vi "VI Tree.vi"   [LabVIEW 2015, in "IT6000C.lvlib"]
doc: "This is the instrument driver for the <INSTRUMENT NAME>. The VI Tree displays all the user-callable VIs of the instrument driver in an organized table."
uses:
  <instrlib>/IT6000C/IT6000C.lvlib
panel:
  # "(c) 2014 <Enter Company Name Here>.  ALL RIGHTS RESERVED."
  # "SEE DIAGRAM\nFOR VI TREE."
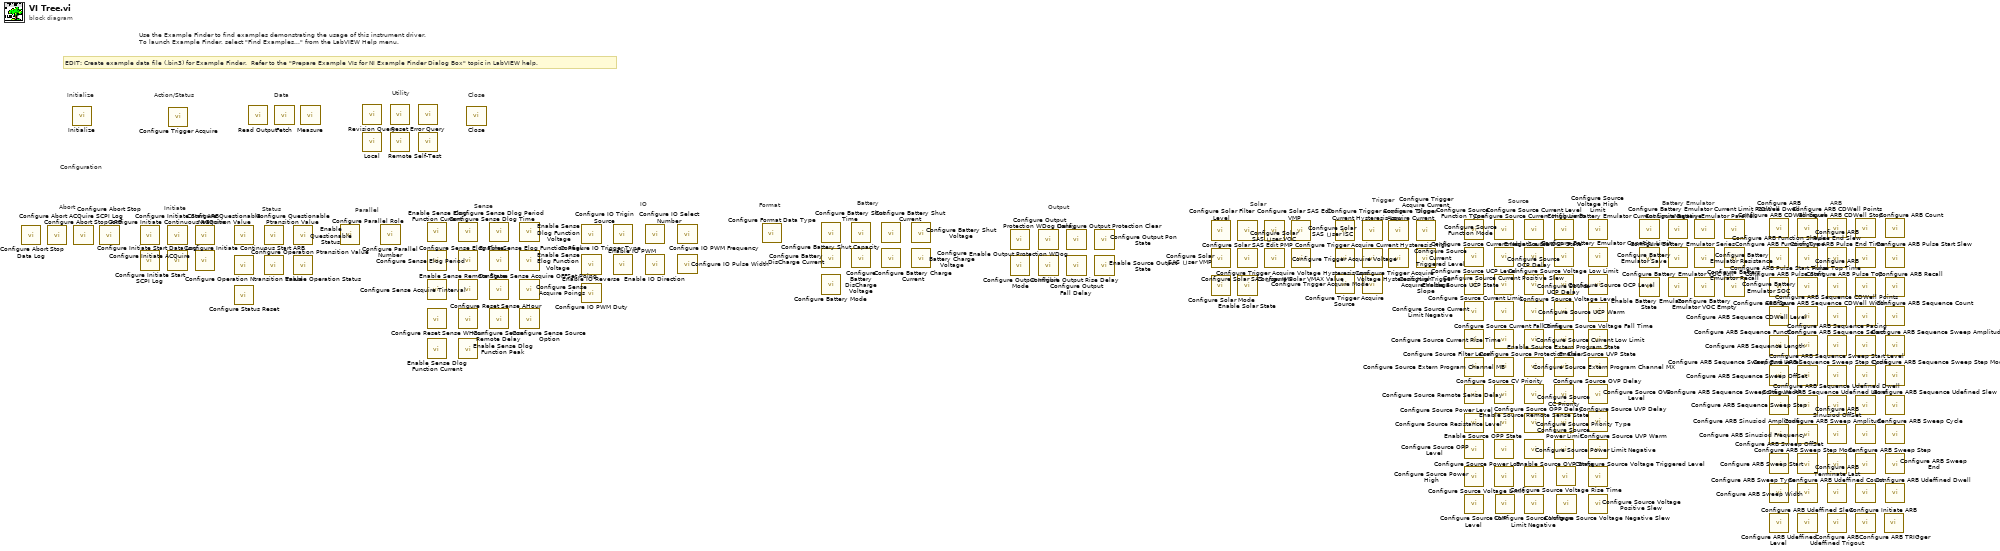
[diagram p0: block diagram]
diagram:
  # "Output"
  # "ARB"
  # "Battery Emulator"
  # "Source"
  # "Trigger"
  # "Solar"
  # "Battery"
  # "Format"
  # "IO"
  # "Sense"
  # "Parallel"
  # "Status"
  # "Initiate"
  # "Abort"
  # "EDIT: Create example data file (.bin3) for Example Finder.  Refer to the \"Prepare Example VIs for NI Example Finder Dialog Box\" topic in LabVIEW help."
  # "Use the Example Finder to find examples demonstrating the usage of this instrument driver.\nTo launch Example Finder, select \"Find Examples...\" from the LabVIEW Help menu."
  # "Configuration"
  # "Utility"
  # "Data"
  # "Action/Status"
  # "Close"
  # "Initialize"
  n1 = call <instrlib>:"Configure Abort Stop Data Log.vi"() -> ()  [unwired: 10 in, 2 out]
  n2 = call <instrlib>:"Configure Abort ACQuire.vi"() -> ()  [unwired: 10 in, 2 out]
  n3 = call <instrlib>:"Initialize.vi"() -> ()  [unwired: 10 in, 2 out]
  n4 = call <instrlib>:"Configure Abort Stop ARB.vi"() -> ()  [unwired: 10 in, 2 out]
  n5 = call <instrlib>:"Configure Abort Stop SCPI Log.vi"() -> ()  [unwired: 10 in, 2 out]
  n6 = call <instrlib>:"Configure Initiate ACQuire.vi"() -> ()  [unwired: 10 in, 2 out]
  n7 = call <instrlib>:"Configure Initiate Start SCPI Log.vi"() -> ()  [unwired: 10 in, 2 out]
  n8 = call <instrlib>:"Configure Initiate Start ARB.vi"() -> ()  [unwired: 10 in, 2 out]
  n9 = call <instrlib>:"Configure Initiate Start Data Log.vi"() -> ()  [unwired: 10 in, 2 out]
  n10 = call <instrlib>:"Configure Trigger Acquire.vi"() -> ()  [unwired: 10 in, 2 out]
  n11 = call <instrlib>:"Configure Initiate Continuous ACQuire.vi"() -> ()  [unwired: 10 in, 2 out]
  n12 = call <instrlib>:"Configure Initiate Continuous Start ARB.vi"() -> ()  [unwired: 10 in, 2 out]
  n13 = call <instrlib>:"Configure Questionable Ntransition Value.vi"() -> ()  [unwired: 10 in, 2 out]
  n14 = call <instrlib>:"Configure Operation Ntransition Value.vi"() -> ()  [unwired: 10 in, 2 out]
  n15 = call <instrlib>:"Configure Status Reset.vi"() -> ()  [unwired: 10 in, 2 out]
  n16 = call <instrlib>:"Read Output.vi"() -> ()  [unwired: 8 in, 4 out]
  n17 = call <instrlib>:"Configure Questionable Ptransition Value.vi"() -> ()  [unwired: 10 in, 2 out]
  n18 = call <instrlib>:"Configure Operation Ptransition Value.vi"() -> ()  [unwired: 10 in, 2 out]
  n19 = call <instrlib>:"Fetch.vi"() -> ()  [unwired: 9 in, 3 out]
  n20 = call <instrlib>:"Enable Questionable Status.vi"() -> ()  [unwired: 10 in, 2 out]
  n21 = call <instrlib>:"Enable Operation Status.vi"() -> ()  [unwired: 10 in, 2 out]
  n22 = call <instrlib>:"Measure.vi"() -> ()  [unwired: 9 in, 3 out]
  n23 = call <instrlib>:"Configure Parallel Role.vi"() -> ()  [unwired: 10 in, 2 out]
  n24 = call <instrlib>:"Revision Query.vi"() -> ()  [unwired: 8 in, 4 out]
  n25 = call <instrlib>:"Local.vi"() -> ()  [unwired: 10 in, 2 out]
  n26 = call <instrlib>:"Configure Parallel Number.vi"() -> ()  [unwired: 10 in, 2 out]
  n27 = call <instrlib>:"Reset.vi"() -> ()  [unwired: 10 in, 2 out]
  n28 = call <instrlib>:"Remote.vi"() -> ()  [unwired: 10 in, 2 out]
  n29 = call <instrlib>:"Error Query.vi"() -> ()  [unwired: 8 in, 4 out]
  n30 = call <instrlib>:"Self-Test.vi"() -> ()  [unwired: 8 in, 4 out]
  n31 = call <instrlib>:"Enable Sense Elog Function Current.vi"() -> ()  [unwired: 10 in, 2 out]
  n32 = call <instrlib>:"Configure Sense Elog Time.vi"() -> ()  [unwired: 10 in, 2 out]
  n33 = call <instrlib>:"Enable Sense Remote State.vi"() -> ()  [unwired: 10 in, 2 out]
  n34 = call <instrlib>:"Configure Reset Sense WHour.vi"() -> ()  [unwired: 10 in, 2 out]
  n35 = call <instrlib>:"Enable Sense Dlog Function Current.vi"() -> ()  [unwired: 10 in, 2 out]
  n36 = call <instrlib>:"Configure Sense Dlog Time.vi"() -> ()  [unwired: 10 in, 2 out]
  n37 = call <instrlib>:"Configure Sense Elog Period.vi"() -> ()  [unwired: 10 in, 2 out]
  n38 = call <instrlib>:"Configure Sense Acquire Tinterval.vi"() -> ()  [unwired: 10 in, 2 out]
  n39 = call <instrlib>:"Configure Reset Sense AHour.vi"() -> ()  [unwired: 10 in, 2 out]
  n40 = call <instrlib>:"Enable Sense Dlog Function Peak.vi"() -> ()  [unwired: 10 in, 2 out]
  n41 = call <instrlib>:"Close.vi"() -> ()  [unwired: 11 in, 1 out]
  n42 = call <instrlib>:"Configure Sense Dlog Period.vi"() -> ()  [unwired: 10 in, 2 out]
  n43 = call <instrlib>:"Enable Sense Elog Function Peak.vi"() -> ()  [unwired: 10 in, 2 out]
  n44 = call <instrlib>:"Configure Sense Acquire OFFSet Poing.vi"() -> ()  [unwired: 10 in, 2 out]
  n45 = call <instrlib>:"Configure Sense Remote Delay.vi"() -> ()  [unwired: 10 in, 2 out]
  n46 = call <instrlib>:"Enable Sense Dlog Function Voltage.vi"() -> ()  [unwired: 10 in, 2 out]
  n47 = call <instrlib>:"Enable Sense Elog Function Voltage.vi"() -> ()  [unwired: 10 in, 2 out]
  n48 = call <instrlib>:"Configure Sense Acquire Poings.vi"() -> ()  [unwired: 10 in, 2 out]
  n49 = call <instrlib>:"Configure Sense Source Option.vi"() -> ()  [unwired: 10 in, 2 out]
  n50 = call <instrlib>:"Configure IO Trigin Source.vi"() -> ()  [unwired: 10 in, 2 out]
  n51 = call <instrlib>:"Enable IO Reverse.vi"() -> ()  [unwired: 10 in, 2 out]
  n52 = call <instrlib>:"Configure IO PWM Duty.vi"() -> ()  [unwired: 10 in, 2 out]
  n53 = call <instrlib>:"Configure IO Trigger Type.vi"() -> ()  [unwired: 10 in, 2 out]
  n54 = call <instrlib>:"Enable IO PWM.vi"() -> ()  [unwired: 10 in, 2 out]
  n55 = call <instrlib>:"Configure IO Select Number.vi"() -> ()  [unwired: 10 in, 2 out]
  n56 = call <instrlib>:"Enable IO Direction.vi"() -> ()  [unwired: 10 in, 2 out]
  n57 = call <instrlib>:"Configure IO PWM Frequency.vi"() -> ()  [unwired: 10 in, 2 out]
  n58 = call <instrlib>:"Configure IO Pulse Width.vi"() -> ()  [unwired: 10 in, 2 out]
  n59 = call <instrlib>:"Configure Format Data Type.vi"() -> ()  [unwired: 10 in, 2 out]
  n60 = call <instrlib>:"Configure Battery Shut Time.vi"() -> ()  [unwired: 10 in, 2 out]
  n61 = call <instrlib>:"Configure Battery DisCharge Current.vi"() -> ()  [unwired: 10 in, 2 out]
  n62 = call <instrlib>:"Configure Battery Mode.vi"() -> ()  [unwired: 10 in, 2 out]
  n63 = call <instrlib>:"Configure Battery Shut Capacity.vi"() -> ()  [unwired: 10 in, 2 out]
  n64 = call <instrlib>:"Configure Battery DisCharge Voltage.vi"() -> ()  [unwired: 10 in, 2 out]
  n65 = call <instrlib>:"Configure Battery Shut Current.vi"() -> ()  [unwired: 10 in, 2 out]
  n66 = call <instrlib>:"Configure Battery Charge Current.vi"() -> ()  [unwired: 10 in, 2 out]
  n67 = call <instrlib>:"Configure Battery Shut Voltage.vi"() -> ()  [unwired: 10 in, 2 out]
  n68 = call <instrlib>:"Configure Battery Charge Voltage.vi"() -> ()  [unwired: 10 in, 2 out]
  n69 = call <instrlib>:"Configure Output Protection WDog Delay.vi"() -> ()  [unwired: 10 in, 2 out]
  n70 = call <instrlib>:"Configure Output Inhibit Mode.vi"() -> ()  [unwired: 10 in, 2 out]
  n71 = call <instrlib>:"Enable Output Protection WDog.vi"() -> ()  [unwired: 10 in, 2 out]
  n72 = call <instrlib>:"Configure Output Rise Delay.vi"() -> ()  [unwired: 10 in, 2 out]
  n73 = call <instrlib>:"Configure Output Protection Clear.vi"() -> ()  [unwired: 10 in, 2 out]
  n74 = call <instrlib>:"Configure Output Fall Delay.vi"() -> ()  [unwired: 10 in, 2 out]
  n75 = call <instrlib>:"Configure Output Pon State.vi"() -> ()  [unwired: 10 in, 2 out]
  n76 = call <instrlib>:"Enable Source Output State.vi"() -> ()  [unwired: 10 in, 2 out]
  n77 = call <instrlib>:"Configure Solar Filter Level.vi"() -> ()  [unwired: 10 in, 2 out]
  n78 = call "Configure Solar SAS Ｕser VMP.vi"() -> ()  [unwired: 10 in, 2 out]
  n79 = call <instrlib>:"Configure Solar Mode.vi"() -> ()  [unwired: 10 in, 2 out]
  n80 = call <instrlib>:"Configure Solar SAS Edit PMP.vi"() -> ()  [unwired: 10 in, 2 out]
  n81 = call "Configure Solar SAS Ｕser IMP.vi"() -> ()  [unwired: 10 in, 2 out]
  n82 = call <instrlib>:"Enable Solar State.vi"() -> ()  [unwired: 10 in, 2 out]
  n83 = call <instrlib>:"Configure Solar SAS Edit VMP.vi"() -> ()  [unwired: 10 in, 2 out]
  n84 = call "Configure Solar SAS Ｕser VOC.vi"() -> ()  [unwired: 10 in, 2 out]
  n85 = call "Configure Solar SAS Ｕser ISC.vi"() -> ()  [unwired: 10 in, 2 out]
  n86 = call <instrlib>:"Configure Solar VMAX Value.vi"() -> ()  [unwired: 10 in, 2 out]
  n87 = call <instrlib>:"Configure Trigger Acquire Current Hysteresis Low.vi"() -> ()  [unwired: 10 in, 2 out]
  n88 = call <instrlib>:"Configure Trigger Acquire Voltage Hysteresis Low.vi"() -> ()  [unwired: 10 in, 2 out]
  n89 = call <instrlib>:"Configure Trigger Acquire Source.vi"() -> ()  [unwired: 10 in, 2 out]
  n90 = call <instrlib>:"Configure Trigger Acquire Current Hysteresis High.vi"() -> ()  [unwired: 10 in, 2 out]
  n91 = call <instrlib>:"Configure Trigger Acquire Voltage Hysteresis High.vi"() -> ()  [unwired: 10 in, 2 out]
  n92 = call <instrlib>:"Configure Trigger Acquire Mode.vi"() -> ()  [unwired: 10 in, 2 out]
  n93 = call <instrlib>:"Configure Trigger Acquire Current.vi"() -> ()  [unwired: 10 in, 2 out]
  n94 = call <instrlib>:"Configure Trigger Acquire Voltage.vi"() -> ()  [unwired: 10 in, 2 out]
  n95 = call <instrlib>:"Configure Trigger Acquire Current Slope.vi"() -> ()  [unwired: 10 in, 2 out]
  n96 = call <instrlib>:"Configure Trigger Acquire Voltage Slope.vi"() -> ()  [unwired: 10 in, 2 out]
  n97 = call <instrlib>:"Configure Source Function Type.vi"() -> ()  [unwired: 10 in, 2 out]
  n98 = call <instrlib>:"Configure Source Current Triggered Level.vi"() -> ()  [unwired: 10 in, 2 out]
  n99 = call <instrlib>:"Configure Source UCP Level.vi"() -> ()  [unwired: 10 in, 2 out]
  n100 = call <instrlib>:"Configure Source Current Limit Negative.vi"() -> ()  [unwired: 10 in, 2 out]
  n101 = call <instrlib>:"Configure Source Current Fall Time.vi"() -> ()  [unwired: 10 in, 2 out]
  n102 = call <instrlib>:"Configure Source Filter Level.vi"() -> ()  [unwired: 10 in, 2 out]
  n103 = call <instrlib>:"Configure Source CV Priority.vi"() -> ()  [unwired: 10 in, 2 out]
  n104 = call <instrlib>:"Configure Source Power Level.vi"() -> ()  [unwired: 10 in, 2 out]
  n105 = call <instrlib>:"Configure Source OPP Level.vi"() -> ()  [unwired: 10 in, 2 out]
  n106 = call <instrlib>:"Configure Source Power High.vi"() -> ()  [unwired: 10 in, 2 out]
  n107 = call <instrlib>:"Configure Source UVP Level.vi"() -> ()  [unwired: 10 in, 2 out]
  n108 = call <instrlib>:"Configure Source Function Mode.vi"() -> ()  [unwired: 10 in, 2 out]
  n109 = call <instrlib>:"Configure Source Current Positive Slew.vi"() -> ()  [unwired: 10 in, 2 out]
  n110 = call <instrlib>:"Enable Source UCP State.vi"() -> ()  [unwired: 10 in, 2 out]
  n111 = call <instrlib>:"Configure Source Current Limit.vi"() -> ()  [unwired: 10 in, 2 out]
  n112 = call <instrlib>:"Configure Source Current Rise Time.vi"() -> ()  [unwired: 10 in, 2 out]
  n113 = call <instrlib>:"Configure Source Extern Program Channel MB.vi"() -> ()  [unwired: 10 in, 2 out]
  n114 = call <instrlib>:"Configure Source Remote Sense Delay.vi"() -> ()  [unwired: 10 in, 2 out]
  n115 = call <instrlib>:"Configure Source Resistance Level.vi"() -> ()  [unwired: 10 in, 2 out]
  n116 = call <instrlib>:"Enable Source OPP State.vi"() -> ()  [unwired: 10 in, 2 out]
  n117 = call <instrlib>:"Configure Source Power Low.vi"() -> ()  [unwired: 10 in, 2 out]
  n118 = call <instrlib>:"Configure Source Voltage Limit.vi"() -> ()  [unwired: 10 in, 2 out]
  n119 = call <instrlib>:"Configure Source Current Level.vi"() -> ()  [unwired: 10 in, 2 out]
  n120 = call <instrlib>:"Configure Source Current Negative Slew.vi"() -> ()  [unwired: 10 in, 2 out]
  n121 = call <instrlib>:"Configure Source OCP Delay.vi"() -> ()  [unwired: 10 in, 2 out]
  n122 = call <instrlib>:"Configure Source UCP Warm.vi"() -> ()  [unwired: 10 in, 2 out]
  n123 = call <instrlib>:"Configure Source Current Low Limit.vi"() -> ()  [unwired: 10 in, 2 out]
  n124 = call <instrlib>:"Configure Source Extern Program Channel MX.vi"() -> ()  [unwired: 9 in, 2 out]
  n125 = call <instrlib>:"Enable Source Remote Sense State.vi"() -> ()  [unwired: 10 in, 2 out]
  n126 = call <instrlib>:"Configure Source Priority Type.vi"() -> ()  [unwired: 10 in, 2 out]
  n127 = call <instrlib>:"Configure Source Power Limit Negative.vi"() -> ()  [unwired: 10 in, 2 out]
  n128 = call <instrlib>:"Enable Source OVP State.vi"() -> ()  [unwired: 10 in, 2 out]
  n129 = call <instrlib>:"Configure Source Voltage Limit Negative.vi"() -> ()  [unwired: 10 in, 2 out]
  n130 = call <instrlib>:"Configure Source Current High Limit.vi"() -> ()  [unwired: 10 in, 2 out]
  n131 = call <instrlib>:"Enable Source OCP State.vi"() -> ()  [unwired: 10 in, 2 out]
  n132 = call <instrlib>:"Configure Source OCP Level.vi"() -> ()  [unwired: 10 in, 2 out]
  n133 = call <instrlib>:"Configure Source UCP Delay.vi"() -> ()  [unwired: 10 in, 2 out]
  n134 = call <instrlib>:"Configure Source Protection Clear.vi"() -> ()  [unwired: 10 in, 2 out]
  n135 = call <instrlib>:"Enable Source Extern Program State.vi"() -> ()  [unwired: 10 in, 2 out]
  n136 = call <instrlib>:"Configure Source OPP Delay.vi"() -> ()  [unwired: 10 in, 2 out]
  n137 = call <instrlib>:"Configure Source CC Priority.vi"() -> ()  [unwired: 10 in, 2 out]
  n138 = call <instrlib>:"Configure Source Power Limit.vi"() -> ()  [unwired: 10 in, 2 out]
  n139 = call <instrlib>:"Configure Source Voltage Rise Time.vi"() -> ()  [unwired: 10 in, 2 out]
  n140 = call <instrlib>:"Configure Source Voltage Negative Slew.vi"() -> ()  [unwired: 10 in, 2 out]
  n141 = call <instrlib>:"Configure Source Voltage High Limit.vi"() -> ()  [unwired: 10 in, 2 out]
  n142 = call <instrlib>:"Configure Source Voltage Low Limit.vi"() -> ()  [unwired: 10 in, 2 out]
  n143 = call <instrlib>:"Configure Source Voltage Level.vi"() -> ()  [unwired: 10 in, 2 out]
  n144 = call <instrlib>:"Configure Source Voltage Fall Time.vi"() -> ()  [unwired: 10 in, 2 out]
  n145 = call <instrlib>:"Enable Source UVP State.vi"() -> ()  [unwired: 10 in, 2 out]
  n146 = call <instrlib>:"Configure Source OVP Delay.vi"() -> ()  [unwired: 10 in, 2 out]
  n147 = call <instrlib>:"Configure Source OVP Level.vi"() -> ()  [unwired: 10 in, 2 out]
  n148 = call <instrlib>:"Configure Source UVP Delay.vi"() -> ()  [unwired: 10 in, 2 out]
  n149 = call <instrlib>:"Configure Source UVP Warm.vi"() -> ()  [unwired: 10 in, 2 out]
  n150 = call <instrlib>:"Configure Source Voltage Triggered Level.vi"() -> ()  [unwired: 10 in, 2 out]
  n151 = call <instrlib>:"Configure Source Voltage Positive Slew.vi"() -> ()  [unwired: 10 in, 2 out]
  n152 = call <instrlib>:"Configure Battery Emulator Capacity Limit.vi"() -> ()  [unwired: 10 in, 2 out]
  n153 = call <instrlib>:"Configure Battery Emulator Series.vi"() -> ()  [unwired: 10 in, 2 out]
  n154 = call <instrlib>:"Enable Battery Emulator State.vi"() -> ()  [unwired: 10 in, 2 out]
  n155 = call <instrlib>:"Configure Battery Emulator Current Limit Negative.vi"() -> ()  [unwired: 10 in, 2 out]
  n156 = call <instrlib>:"Configure Battery Emulator Save.vi"() -> ()  [unwired: 10 in, 2 out]
  n157 = call <instrlib>:"Configure Battery Emulator VOC Full.vi"() -> ()  [unwired: 10 in, 2 out]
  n158 = call <instrlib>:"Configure Battery Emulator Current Limit Positive.vi"() -> ()  [unwired: 10 in, 2 out]
  n159 = call <instrlib>:"Configure Battery Emulator Resistance.vi"() -> ()  [unwired: 10 in, 2 out]
  n160 = call <instrlib>:"Configure Battery Emulator VOC Empty.vi"() -> ()  [unwired: 10 in, 2 out]
  n161 = call <instrlib>:"Configure Battery Emulator Parallel.vi"() -> ()  [unwired: 10 in, 2 out]
  n162 = call <instrlib>:"Configure Battery Emulator Recall.vi"() -> ()  [unwired: 10 in, 2 out]
  n163 = call <instrlib>:"Configure Battery Emulator SOC.vi"() -> ()  [unwired: 10 in, 2 out]
  n164 = call <instrlib>:"Configure ARB CDWell Dwell.vi"() -> ()  [unwired: 10 in, 2 out]
  n165 = call <instrlib>:"Configure ARB Function Shape.vi"() -> ()  [unwired: 10 in, 2 out]
  n166 = call <instrlib>:"Configure ARB Pulse Start Time.vi"() -> ()  [unwired: 10 in, 2 out]
  n167 = call <instrlib>:"Configure ARB Save.vi"() -> ()  [unwired: 10 in, 2 out]
  n168 = call <instrlib>:"Configure ARB Sequence Function.vi"() -> ()  [unwired: 10 in, 2 out]
  n169 = call <instrlib>:"Configure ARB Sequence Sweep End Level.vi"() -> ()  [unwired: 10 in, 2 out]
  n170 = call <instrlib>:"Configure ARB Sequence Sweep Step Width.vi"() -> ()  [unwired: 10 in, 2 out]
  n171 = call <instrlib>:"Configure ARB Sinusiod Amplitude.vi"() -> ()  [unwired: 10 in, 2 out]
  n172 = call <instrlib>:"Configure ARB Sweep OffSet.vi"() -> ()  [unwired: 10 in, 2 out]
  n173 = call <instrlib>:"Configure ARB Sweep Type.vi"() -> ()  [unwired: 10 in, 2 out]
  n174 = call <instrlib>:"Configure ARB Udeffined Level.vi"() -> ()  [unwired: 10 in, 2 out]
  n175 = call <instrlib>:"Configure ARB CDWell Level.vi"() -> ()  [unwired: 10 in, 2 out]
  n176 = call <instrlib>:"Configure ARB Function Type.vi"() -> ()  [unwired: 10 in, 2 out]
  n177 = call <instrlib>:"Configure ARB Pulse Start.vi"() -> ()  [unwired: 10 in, 2 out]
  n178 = call <instrlib>:"Configure ARB Sequence CDWell Level.vi"() -> ()  [unwired: 10 in, 2 out]
  n179 = call <instrlib>:"Configure ARB Sequence Length.vi"() -> ()  [unwired: 10 in, 2 out]
  n180 = call <instrlib>:"Configure ARB Sequence Sweep OffSet.vi"() -> ()  [unwired: 10 in, 2 out]
  n181 = call <instrlib>:"Configure ARB Sequence Sweep Step.vi"() -> ()  [unwired: 10 in, 2 out]
  n182 = call <instrlib>:"Configure ARB Sinusiod Frequency.vi"() -> ()  [unwired: 10 in, 2 out]
  n183 = call <instrlib>:"Configure ARB Sweep Start.vi"() -> ()  [unwired: 10 in, 2 out]
  n184 = call <instrlib>:"Configure ARB Sweep Width.vi"() -> ()  [unwired: 10 in, 2 out]
  n185 = call <instrlib>:"Configure ARB Udeffined Slew.vi"() -> ()  [unwired: 10 in, 2 out]
  n186 = call <instrlib>:"Configure ARB CDWell Points.vi"() -> ()  [unwired: 10 in, 2 out]
  n187 = call <instrlib>:"Configure ARB Pulse End Slew.vi"() -> ()  [unwired: 10 in, 2 out]
  n188 = call <instrlib>:"Configure ARB Pulse Top Time.vi"() -> ()  [unwired: 10 in, 2 out]
  n189 = call <instrlib>:"Configure ARB Sequence CDWell Points.vi"() -> ()  [unwired: 10 in, 2 out]
  n190 = call <instrlib>:"Configure ARB Sequence Pacing.vi"() -> ()  [unwired: 10 in, 2 out]
  n191 = call <instrlib>:"Configure ARB Sequence Sweep Start Level.vi"() -> ()  [unwired: 10 in, 2 out]
  n192 = call <instrlib>:"Configure ARB Sequence Udefined Dwell.vi"() -> ()  [unwired: 10 in, 2 out]
  n193 = call <instrlib>:"Configure ARB Sinusiod OffSet.vi"() -> ()  [unwired: 10 in, 2 out]
  n194 = call <instrlib>:"Configure ARB Sweep Step Mode.vi"() -> ()  [unwired: 10 in, 2 out]
  n195 = call <instrlib>:"Configure ARB Terminate Last.vi"() -> ()  [unwired: 10 in, 2 out]
  n196 = call <instrlib>:"Configure ARB Udeffined Trigout.vi"() -> ()  [unwired: 10 in, 2 out]
  n197 = call <instrlib>:"Configure ARB CDWell Stop.vi"() -> ()  [unwired: 10 in, 2 out]
  n198 = call <instrlib>:"Configure ARB Pulse End Time.vi"() -> ()  [unwired: 10 in, 2 out]
  n199 = call <instrlib>:"Configure ARB Pulse Top.vi"() -> ()  [unwired: 10 in, 2 out]
  n200 = call <instrlib>:"Configure ARB Sequence CDWell Width.vi"() -> ()  [unwired: 10 in, 2 out]
  n201 = call <instrlib>:"Configure ARB Sequence Select.vi"() -> ()  [unwired: 10 in, 2 out]
  n202 = call <instrlib>:"Configure ARB Sequence Sweep Step Cycle.vi"() -> ()  [unwired: 10 in, 2 out]
  n203 = call <instrlib>:"Configure ARB Sequence Udefined Level.vi"() -> ()  [unwired: 10 in, 2 out]
  n204 = call <instrlib>:"Configure ARB Sweep Amplitude.vi"() -> ()  [unwired: 10 in, 2 out]
  n205 = call <instrlib>:"Configure ARB Sweep Step.vi"() -> ()  [unwired: 10 in, 2 out]
  n206 = call <instrlib>:"Configure ARB Udeffined Count.vi"() -> ()  [unwired: 10 in, 2 out]
  n207 = call <instrlib>:"Configure Initiate ARB.vi"() -> ()  [unwired: 10 in, 2 out]
  n208 = call <instrlib>:"Configure ARB TRIGger.vi"() -> ()  [unwired: 12 in]
  n209 = call <instrlib>:"Configure ARB Count.vi"() -> ()  [unwired: 10 in, 2 out]
  n210 = call <instrlib>:"Configure ARB Pulse Start Slew.vi"() -> ()  [unwired: 10 in, 2 out]
  n211 = call <instrlib>:"Configure ARB Recall.vi"() -> ()  [unwired: 10 in, 2 out]
  n212 = call <instrlib>:"Configure ARB Sequence Count.vi"() -> ()  [unwired: 10 in, 2 out]
  n213 = call <instrlib>:"Configure ARB Sequence Sweep Amplitude.vi"() -> ()  [unwired: 10 in, 2 out]
  n214 = call <instrlib>:"Configure ARB Sequence Sweep Step Mode.vi"() -> ()  [unwired: 10 in, 2 out]
  n215 = call <instrlib>:"Configure ARB Sequence Udefined Slew.vi"() -> ()  [unwired: 10 in, 2 out]
  n216 = call <instrlib>:"Configure ARB Sweep Cycle.vi"() -> ()  [unwired: 10 in, 2 out]
  n217 = call <instrlib>:"Configure ARB Sweep End.vi"() -> ()  [unwired: 10 in, 2 out]
  n218 = call <instrlib>:"Configure ARB Udeffined Dwell.vi"() -> ()  [unwired: 10 in, 2 out]
